vi "macro_Digital_And.vi"   [LabVIEW 2019, in "Trajectory_Library.lvlib"]
uses:
  Trajectory_Library.lvlib
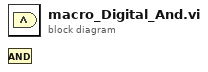
[diagram p0: block diagram]
diagram:
  n1 = And() -> ()  [unwired: 2 in, 1 out]
